vi "Vision Processing.vi"(4 "Camera Settings":T2={"fps"=15, "compression"=5, "Image Size"=enum."320x240"}) -> ()   [LabVIEW 2013]
doc: "This VI runs in parallel to other tasks. It gets images from the camera, processes them for color or shape and use that information to affect robot behavior."
uses:
  <vilib>/Rock Robotics/WPI/Camera/WPI_CameraSettings Read MJPG.ctl
  <vilib>/Rock Robotics/WPI/Camera/WPI_CameraImageSize.ctl
  Robot Global Data.vi
panel:
  out "Image":T1(plugin-control)
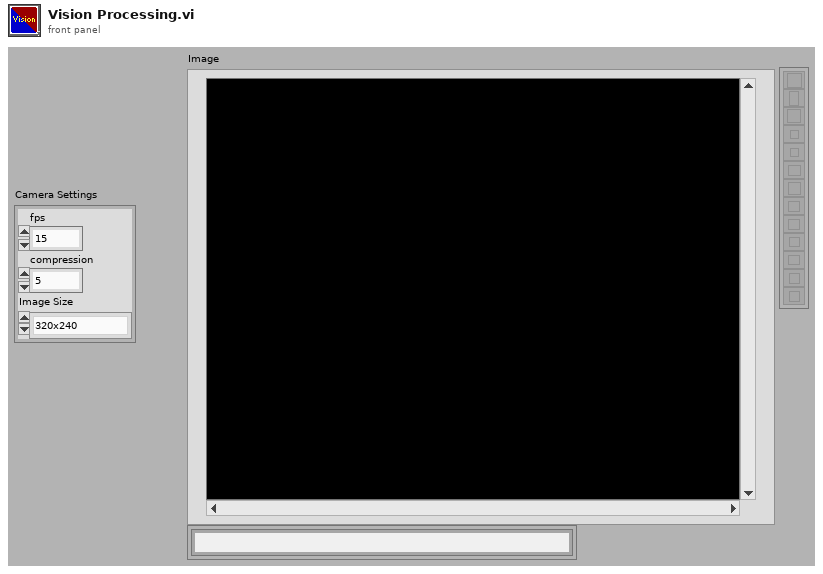
[diagram p1: front panel]
types:
  T1 = typedef "IMAQ Image.ctl" = refnum<image>
  T2 = typedef "WPI_CameraSettings Read MJPG.ctl" = cluster{"fps":i32, "compression":i32, "Image Size":T3}
  T3 = typedef "WPI_CameraImageSize.ctl" = enum16{"640x480", "320x240", "160x120"}
  T4 = typedef "Image Type" = u32
  T5 = cluster{"Hue":cluster{dbl, dbl}, "Sat":cluster{dbl, dbl}, "Val":cluster{dbl, dbl}}
  T6 = cluster{"Horizontal":bool, "Aspect Score":dbl, "Rect Score":dbl, cluster{"Left":dbl, "Top":dbl, "Right":dbl, "Bottom":dbl}, "Equiv H":dbl, "Equiv V":dbl}[]
  T7 = typedef "TargetType.ctl" = enum16{"Not Hot", "Hot"}
  T8 = cluster{"Scores":cluster{"Total":dbl, "Left":dbl, "Right":dbl, "Ratio":dbl, "Vertical":dbl, "index":i32, "State":T7}, "Verticals":cluster{"Horizontal?":bool, "Aspect Score":dbl, "Rect Score":dbl, cluster{"Left":dbl, "Top":dbl, "Right":dbl, "Bottom":dbl}, "Equiv H":dbl, "Equiv V":dbl}, "Horizontals":cluster{"Horizontal?":bool, "Aspect Score":dbl, "Rect Score":dbl, cluster{"Left":dbl, "Top":dbl, "Right":dbl, "Bottom":dbl}, "Equiv H":dbl, "Equiv V":dbl}, "Validated":bool}[]
  T9 = cluster{"Scores":cluster{"Total":dbl, "Left":dbl, "Right":dbl, "Ratio":dbl, "Vertical":dbl, "index":i32, "State":T7}, "Verticals":cluster{"Horizontal?":bool, "Aspect Score":dbl, "Rect Score":dbl, cluster{"Left":dbl, "Top":dbl, "Right":dbl, "Bottom":dbl}, "Equiv H":dbl, "Equiv V":dbl}, "Horizontals":cluster{"Horizontal?":bool, "Aspect Score":dbl, "Rect Score":dbl, cluster{"Left":dbl, "Top":dbl, "Right":dbl, "Bottom":dbl}, "Equiv H":dbl, "Equiv V":dbl}, "Distance (ft)":dbl, "Target Center (-1 to 1)":cluster{"X":dbl, "Y":dbl}}[]
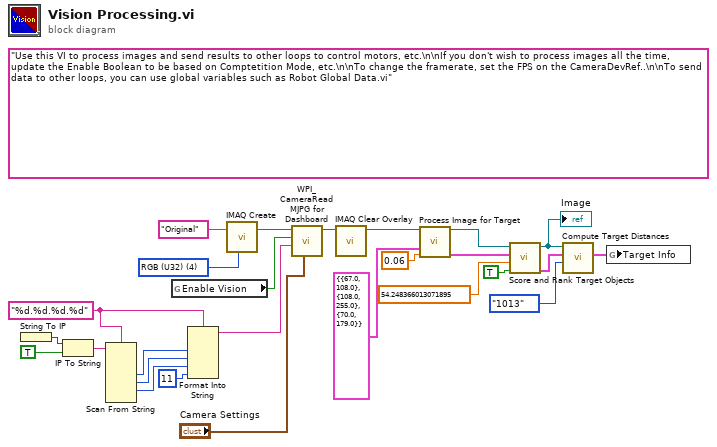
[diagram p0: block diagram]
diagram:
  w18 = T4 4 items=["Grayscale (U8)", "Grayscale (I16)", "Grayscale (SGL)", "Complex (CSG)", "RGB (U32)", "HSL (U32)", "RGB (U64)", "Grayscale (U16)"] ("Image Type")
  w19 = "%d.%d.%d.%d" ("format string")
  (unwired) "Use this VI to process images and send results to other loops to control motors, etc.\n\nIf you don't wish to process images all the time, update the Enable Boolean to be based on Comptetition Mode, etc.\n\nTo change the framerate, set the FPS on the CameraDevRef..\n\nTo send data to other loops, you can use global variables such as Robot Global Data.vi"
  n1 = String To IP() -> (0:w26:u32)  [unwired: 1 in]
  n2 = IP To String(1:TRUE ("dot notation? (F)"), 2:w26) -> (0:w24:string)
  n3 = Scan From String(format string=w19, input string=w24) -> (output 1=w23:i32, output 2=w22:i32, output 3=w21:i32)  [unwired: 7 in, 3 out]
  n4 = global read "Robot Global Data.vi" "Enable Vision"() -> (w1:bool)
  n5 = Format Into String(format string=w19, w23, w22, w21, 11 ("Compression")) -> (resulting string=w15:string)  [unwired: 2 in, 1 out]
  n6 = call "IMAQ Create"("Image Name"="Original", "Image Type"=w18) -> ("New Image"=w16:T1)  [unwired: 3 in, 1 out]
  n7 = call <vilib>:"WPI_CameraRead MJPG for Dashboard.vi"("Camera Settings"="Camera Settings", "Camera IP"=w15, "Enable"=w1, "Refnum in"=w16) -> ("Refnum out"=w13:T1)  [unwired: 4 in, 3 out]
  n8 = call "IMAQ Clear Overlay"("Image"=w13) -> ("Image Out"=w12:T1)  [unwired: 9 in, 1 out]
  n9 = call "Process Image for Target.vi"("Src Image"=w12, "Color Components"=T5 {"Hue"={67.0, 108.0}, "Sat"={108.0, 255.0}, "Val"={70.0, 179.0}}, "Area Cutoff %"=0.06 ("Area Size Limit %")) -> ("Src Image Out"=w2:T1, "Particles"=w6:T6)  [unwired: 10 in, 1 out]
  n10 = call "Score and Rank Target Objects.vi"("Annotate"=TRUE, "Score Limit"=54.248366013071895 ("Score Cutoff"), "Particles"=w6, "Image in"=w2) -> ("Target Info"=w9:T8, "Annotated Image"=w3:T1)  [unwired: 6 in]
  "Image" <- w3
  n11 = call "Compute Target Distances.vi"("Camera Type"=enum16{"206", "1011", "1013"}."1013", "Target Info"=w9, "Image in"=w3) -> ("Target Info"=w8:T9)  [unwired: 6 in, 2 out]
  n12 = global write "Robot Global Data.vi" "Target Info"(w8) -> ()
